vi "Tx FIFOs.vi"(0 "rx.fifo":refnum<k21>="tx 0.fifo", 1 "rx.data sink":enum16{"SFP Port 0", "SFP Port 1", "Host"}(ring)=enum."SFP Port 1", 5 "rx.host fifo":refnum<k21>="tx 0.host fifo", 7 "rx.sfp fifo":refnum<k21>="tx 0sfp 0 fifo") -> ()   [LabVIEW 2016]
uses:
  <vilib>/rvi/DataTransferAndStorage/Container/Common/niFpgaContainerExecOnDevCompGetState.vi
  <vilib>/rvi/Emulation/niFpgaEmulationIsFPGAContextNoSignature.vi
  <vilib>/rvi/Emulation/niFpgaSctlEmulationGetInTimedLoop.vi
  <vilib>/rvi/errors/niFpgaSetErrorForExecOnDevCompSimple.vi
  <vilib>/rvi/eio/common/nirviEmuReportErrorAndStop.vi
  <vilib>/rvi/DataTransferAndStorage/Container/Common/niFpgaContainerGetUniqueNameForEmu.vi
  <vilib>/rvi/FIFO/Fifo_Resource/nirvififoEmulationSetSize.vi
  <vilib>/rvi/FIFO/Fifo_Resource/nirviFifoEmulationQueueMgr.vi
  <instcachedir>/0/nirviFifoEmulationQueueMgr_E5CAEC123FF24DC58D834DCA3CDAA9B5.lvgen/nirviFifoEmulationQueueMgr_E5CAEC123FF24DC58D834DCA3CDAA9B5_003.vi
  <vilib>/rvi/FIFO/Fifo_Resource/nirvififoEmulationDetermineInputValidOut.vi
  <vilib>/rvi/FIFO/Fifo_Resource/nirvififoEmulationCreateLock.vi
  <vilib>/rvi/Emulation/niFpgaProcessEmulError.vi
  <vilib>/rvi/FIFO/Fifo_Resource/nirvififoEmulationObtainLock.vi
  <vilib>/rvi/FIFO/Fifo_Resource/nirvififoEmulationReleaseLock.vi
  <vilib>/rvi/occurrence/nirviWaitOnOccurrenceBase.vi
  <vilib>/rvi/errors/nirviReportUnexpectedCaseInternalError.vi
  <vilib>/rvi/errors/nirviReportUnexpectedCaseInternalError (U32).vi
  <vilib>/Utility/error.llb/Clear Errors.vi
  <vilib>/rvi/interface/RandomDataEmulation/niFpgaRandomDataHandleErrors.vi
  <instcachedir>/0/nirviFifoEmulationQueueMgr_E5CAEC123FF24DC58D834DCA3CDAA9B5.lvgen/nirviFifoEmulationQueueMgr_E5CAEC123FF24DC58D834DCA3CDAA9B5_004.vi
  <vilib>/rvi/DataTransferAndStorage/Container/XNode/niFpgaContainer.xnode
  <vilib>/rvi/FIFO/Fifo_Resource/niFpgaFifoEmulationRefIn.vi
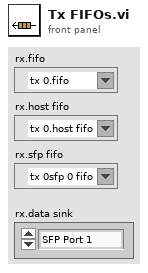
[diagram p1: front panel]
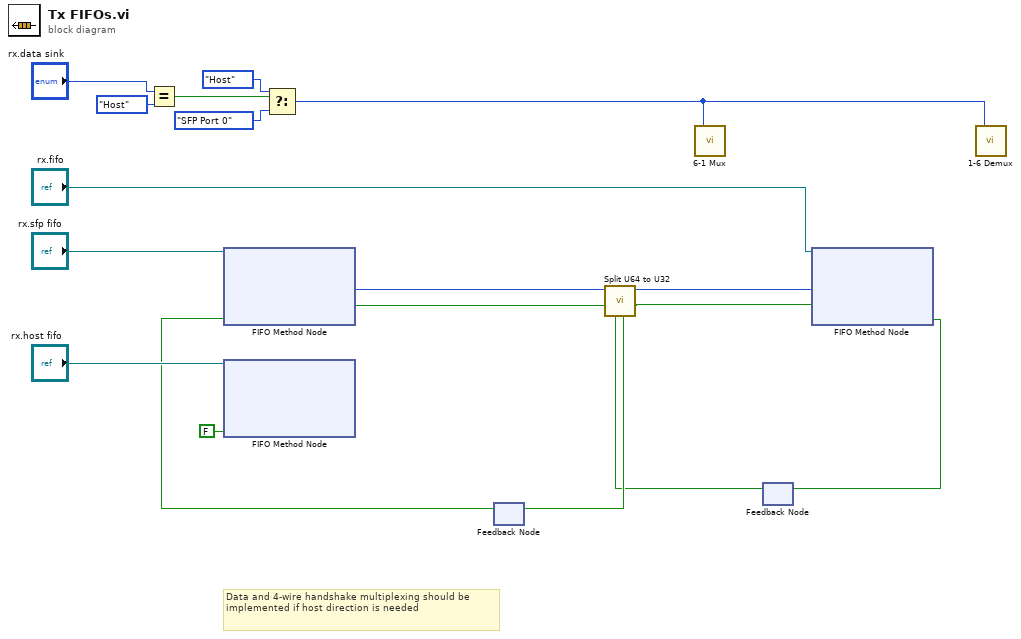
[diagram p0: block diagram]
diagram:
  # "Data and 4-wire handshake multiplexing should be implemented if host direction is needed"
  n1 = Equal?(x="rx.data sink", y=enum16{"SFP Port 0", "SFP Port 1", "Host"}."Host") -> (x = y?=w17:bool)
  n2 = xnode ("FIFO Method Node")("Ready for Output"=FALSE, "FIFO In"="rx.host fifo") -> ()  [unwired: 3 out]
  n3 = Select(t=enum16{"SFP Port 0", "SFP Port 1", "Host"}."Host" ("y"), s=w17, f=enum16{"SFP Port 0", "SFP Port 1", "Host"}."SFP Port 0" ("y")) -> (s? t:f=w10:enum16{"SFP Port 0", "SFP Port 1", "Host"})
  n4 = feedback #1() -> (w7:bool)  [unwired: 1 in]
  n5 = xnode ("FIFO Method Node")("Ready for Output"=w7, "FIFO In"="rx.sfp fifo") -> ("Element"=w6:u64, "Output Valid"=w3:bool)  [unwired: 1 out]
  n6 = call "6-1 Mux.vi"("select"=w10) -> ()  [unwired: 18 in, 1 out]
  n7 = feedback #2() -> (w1:bool)  [unwired: 1 in]
  n8 = call "Split U64 to U32.vi"("ready for output (T)"=w1, "input valid"=w3, "data in"=w6) -> ("output valid"=w4:bool, "data out"=w5:u32, "ready for input"=w2:bool)  [unwired: 6 in]
  n9 = feedback-in #1(w2) -> ()
  n10 = xnode ("FIFO Method Node")("Element"=w5, "Input Valid"=w4, "FIFO In"="rx.fifo") -> ("Ready for Input"=w9:bool)  [unwired: 1 out]
  n11 = feedback-in #2(w9) -> ()
  n12 = call "1-6 Demux.vi"("select"=w10) -> ()  [unwired: 13 in, 6 out]
